vi "Trabajoarreglo1.vi"() -> ()   [LabVIEW 2020]
panel:
  out "Dato2":u8[](array[numeric]) format="%.0x"
  out "Dato1":u8[](array[numeric]) format="%.0x"
  out "RF data":u8[](array[numeric]) format="%.0x"
  out "Tam.Arreglo":i32
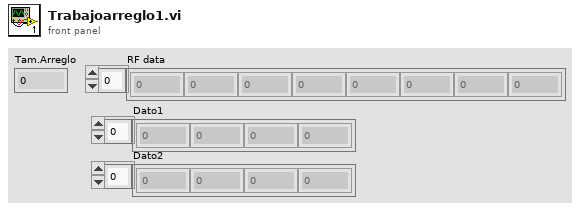
[diagram p1: front panel]
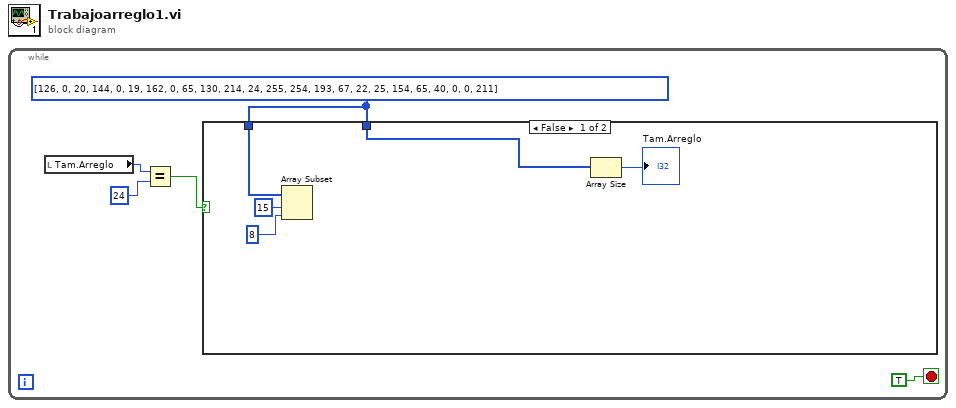
[diagram p0: block diagram]
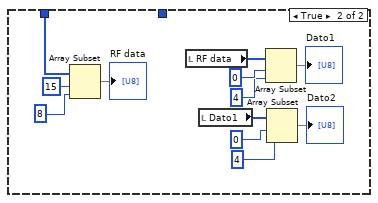
[diagram p2: hidden frame]
diagram:
  n1 = while {
    stop <- TRUE stop-if-true
    w1 = u8[] [126, 0, 20, 144, 0, 19, 162, 0, 65, 130, 214, 24, 255, 254, 193, 67, 22, 25, 154, 65, 40, 0, 0, 211]
    n2 = local read "Tam.Arreglo"() -> (w4:i32)
    n3 = Equal?(x=w4, y=24) -> (x = y?=w2:bool)
    n4 = case shown="False" w2 {
      tunnel: w1 -> [w7 w22]
      tunnel: w1 -> [w10 _]
      frame False {
        n5 = Array Subset(array=w7, index=15, length=8) -> ()  [unwired: 1 out]
        n6 = Array Size(array=w10) -> (size(s)=→"Tam.Arreglo":i32)
      }
      frame True {
        n7 = Array Subset(array=w22, index=15, length=8) -> (→"RF data":u8[])
        n8 = local read "RF data"() -> (w19:u8[])
        n9 = local read "Dato1"() -> (w11:u8[])
        n10 = Array Subset(array=w19, index=0, length=4) -> (→"Dato1":u8[])
        n11 = Array Subset(array=w11, index=0, length=4) -> (→"Dato2":u8[])
      }
    }
  }
